vi "ConvTemp.vi"(8 "error constant":errorcluster, 11 "DataIn":i32) -> (0 "error constant 2":errorcluster, 3 "Temperature":dbl)   [LabVIEW 2022 SP3]
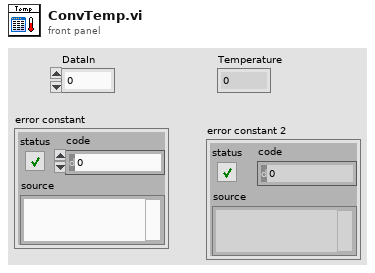
[diagram p1: front panel]
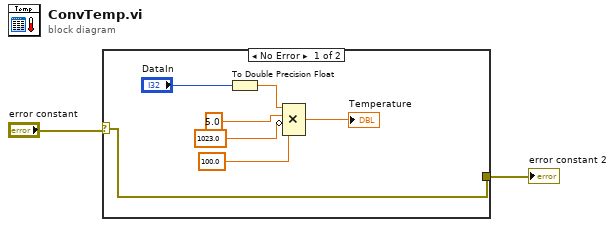
[diagram p0: block diagram]
diagram:
  n1 = case shown="No Error" "error constant" {
    selector: "error constant" -> [w4 w10]
    tunnel: [w4 w10] -> w1
    frame No Error {
      n2 = To Double Precision Float(number="DataIn") -> (double precision float=w3:dbl)
      n3 = Compound Arithmetic op=MULTIPLY(w3, 5.0, invert 1023.0, 100.0) -> (→"Temperature":dbl)
    }
    frame Error {
    }
  }
  "error constant 2" <- w1
